vi "myRIO_BRig_RT_dataCurrent_nENL1.vi"() -> (2 "output_nENL1":i32)   [LabVIEW 2014]
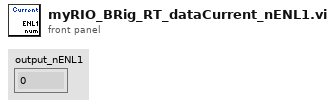
[diagram p1: front panel]
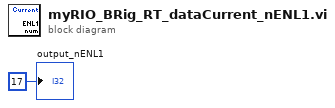
[diagram p0: block diagram]
diagram:
  "output_nENL1" <- 17 ("output_iBlock")
